vi "Update Map Yaml.vi"(8 "error in (no error)":errorcluster, 10 "Map Yaml":T1, 11 "Yaml Model in":refnum<class "Yaml Model.lvclass">) -> (0 "error out":errorcluster, 3 "Yaml Model out":refnum<class "Yaml Model.lvclass">)   [LabVIEW 2020, in "Yaml Model.lvlib" / "Yaml Model.lvclass"]
uses:
  Yaml Model.lvclass
  Yaml Model.lvclass/Yaml Model.ctl
panel:
  # "NOTICE -- YOU MUST LEAVE THIS NOTICE IN PLACE.\n\nCopyright (c) 2017, LIANG LIU Shawn.Liu.cn@gmail.com\nAll rights reserved.\n\nRedistribution and use in source and binary forms, with or without modification, are permitted provided that the following conditions are met:\n-Redistributions of source code must retain the above copyright notice, this list of conditions and the following disclaimer.\n-Redistributions in binary form must reproduce the above copyright notice, this list of conditions and the following disclaimer in the documentation and/or other materials provided with the distribution.\n-Neither the name of the eLp nor the names of its contributors may be used to endorse or promote products derived from this software without specific prior written permission.\n\nTHIS SOFTWARE IS PROVIDED BY THE COPYRIGHT HOLDERS AND CONTRIBUTORS \"AS IS\" AND ANY EXPRESS OR IMPLIED WARRANTIES, INCLUDING, BUT NOT LIMITED TO, THE IMPLIED WARRANTIES OF MERCHANTABILITY AND FITNESS FOR A PARTICULAR PURPOSE ARE DISCLAIMED. IN NO EVENT SHALL THE COPYRIGHT HOLDER OR CONTRIBUTORS BE LIABLE FOR ANY DIRECT, INDIRECT, INCIDENTAL, SPECIAL, EXEMPLARY, OR CONSEQUENTIAL DAMAGES (INCLUDING, BUT NOT LIMITED TO, PROCUREMENT OF SUBSTITUTE GOODS OR SERVICES; LOSS OF USE, DATA, OR PROFITS; OR BUSINESS INTERRUPTION) HOWEVER CAUSED AND ON ANY THEORY OF LIABILITY, WHETHER IN CONTRACT, STRICT LIABILITY, OR TORT (INCLUDING NEGLIGENCE OR OTHERWISE) ARISING IN ANY WAY OUT OF THE USE OF THIS SOFTWARE, EVEN IF ADVISED OF THE POSSIBILITY OF SUCH DAMAGE."
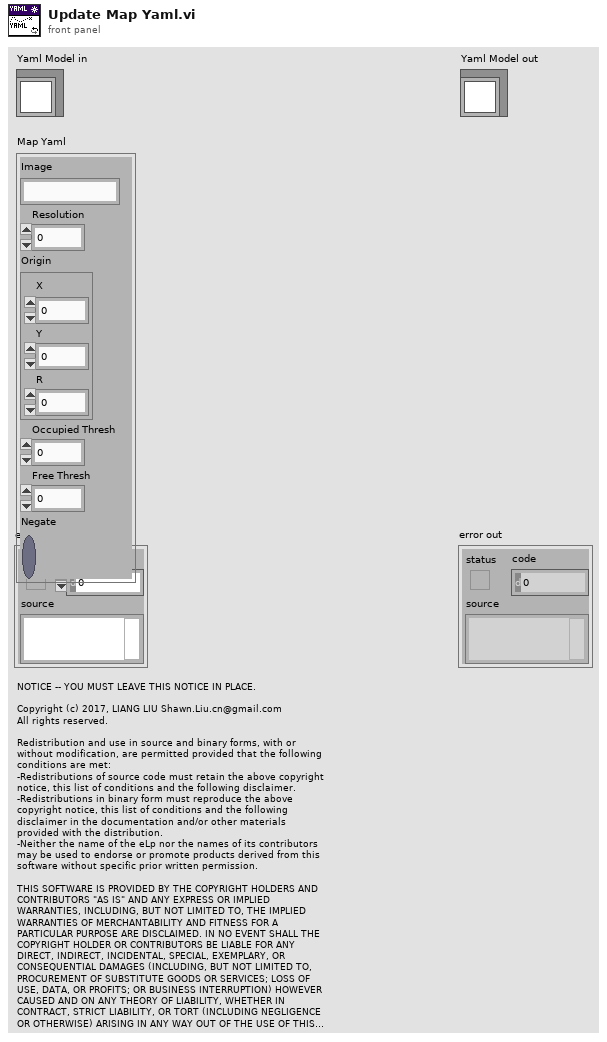
[diagram p1: front panel]
types:
  T1 = cluster{"Image":string, "Resolution":dbl, "Origin":cluster{"X":dbl, "Y":dbl, "R":dbl}, "Occupied Thresh":dbl, "Free Thresh":dbl, "Negate":bool}
  T2 = enum8{"Enabled", "Disabled", "Disabled and Grayed Out"}
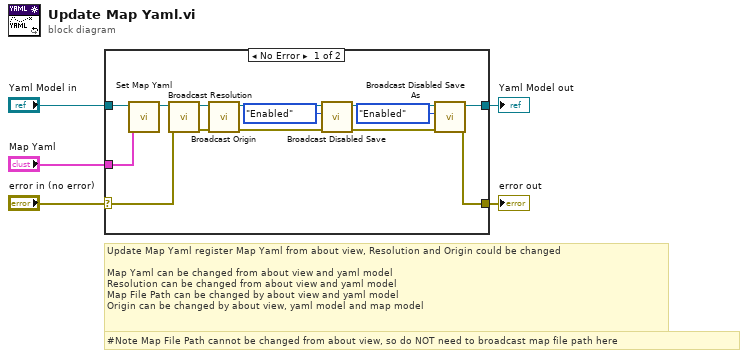
[diagram p0: block diagram]
diagram:
  # "#Note Map File Path cannot be changed from about view, so do NOT need to broadcast map file path here"
  # "Update Map Yaml register Map Yaml from about view, Resolution and Origin could be changed\n\nMap Yaml can be changed from about view and yaml model\nResolution can be changed from about view and yaml model\nMap File Path can be changed by about view and yaml model\nOrigin can be changed by about view, yaml model and map model"
  n1 = case shown="No Error" "error in (no error)" {
    selector: "error in (no error)" -> [w19 w21]
    tunnel: "Yaml Model in" -> [w18 w20]
    tunnel: "Map Yaml" -> [w17 _]
    tunnel: [w16 w20] -> w2
    tunnel: [w15 w21] -> w1
    frame No Error {
      n2 = call "Set Map Yaml.vi"("Map Yaml"=w17, "Yaml Model in"=w18) -> ("Yaml Model out"=w8:refnum<class "Yaml Model.lvclass">)  [unwired: 9 in]
      n3 = call "Broadcast Resolution.vi"("error in (no error)"=w19, "Yaml Model in"=w8) -> ("error out"=w6:errorcluster, "Yaml Model out"=w7:refnum<class "Yaml Model.lvclass">)  [unwired: 8 in]
      n4 = call "Broadcast Origin.vi"("error in (no error)"=w6, "Yaml Model in"=w7) -> ("error out"=w10:errorcluster, "Yaml Model out"=w9:refnum<class "Yaml Model.lvclass">)  [unwired: 8 in]
      n5 = call "Broadcast Disabled Save.vi"("error in (no error)"=w10, "Disabled Save"=T2."Enabled", "Yaml Model in"=w9) -> ("error out"=w11:errorcluster, "Yaml Model out"=w14:refnum<class "Yaml Model.lvclass">)  [unwired: 7 in]
      n6 = call "Broadcast Disabled Save As.vi"("error in (no error)"=w11, "Disabled Save As"=T2."Enabled", "Yaml Model in"=w14) -> ("error out"=w15:errorcluster, "Yaml Model out"=w16:refnum<class "Yaml Model.lvclass">)  [unwired: 7 in]
    }
    frame Error {
    }
  }
  "error out" <- w1
  "Yaml Model out" <- w2
